vi "PIDControllers (SubVI).vi"(0 "HMI-10HIC200":dbl, 1 "HMI-10LIC200_MA":bool, 2 "BPCS-10LI200":dbl, 3 "HMI-10LIC200-SP":dbl, 5 "HMI-10LIC200-KPID":dbl[](array[numeric]), 7 "HMI-10TIC100-SP":dbl, 9 "BPCS-10TI100":dbl, 11 "HMI-10HIC300":dbl, 12 "HMI-10TIC100_MA":bool, 13 "HMI-10HIC100":dbl, 14 "HMI-10TIC100-KPID":dbl[](array[numeric]), 15 "BPCS-FJ":dbl) -> (4 "BPCS-10Y200":dbl format="%.2f", 6 "BPCS-SIM-TX-ARRAY":dbl[](array[numeric]), 8 "BPCS-10AY300":dbl, 10 "BPCS-10TY100":dbl format="%.2f")   [LabVIEW 2018]
uses:
  <vilib>/addons/control/pid/pid.llb/PID Advanced (DBL).vi
  <vilib>/addons/control/pid/NI_PID_pid.lvlib
panel:
  out "dt out (s)":dbl format="%.3f"
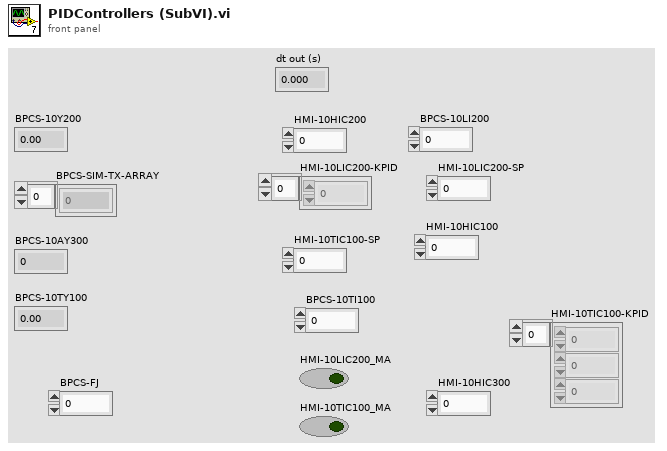
[diagram p1: front panel]
types:
  T1 = cluster{"proportional gain (Kc)":dbl, "integral time (Ti, min)":dbl, "derivative time (Td, min)":dbl}
  T2 = cluster{"HMI-10TIC100-KPID[0]":dbl, "HMI-10TIC100-KPID[1]":dbl, "HMI-10TIC100-KPID[2]":dbl}
  T3 = cluster{"HMI-10LIC200-KPID[0]":dbl, "HMI-10LIC200-KPID[1]":dbl, "HMI-10LIC200-KPID[2]":dbl}
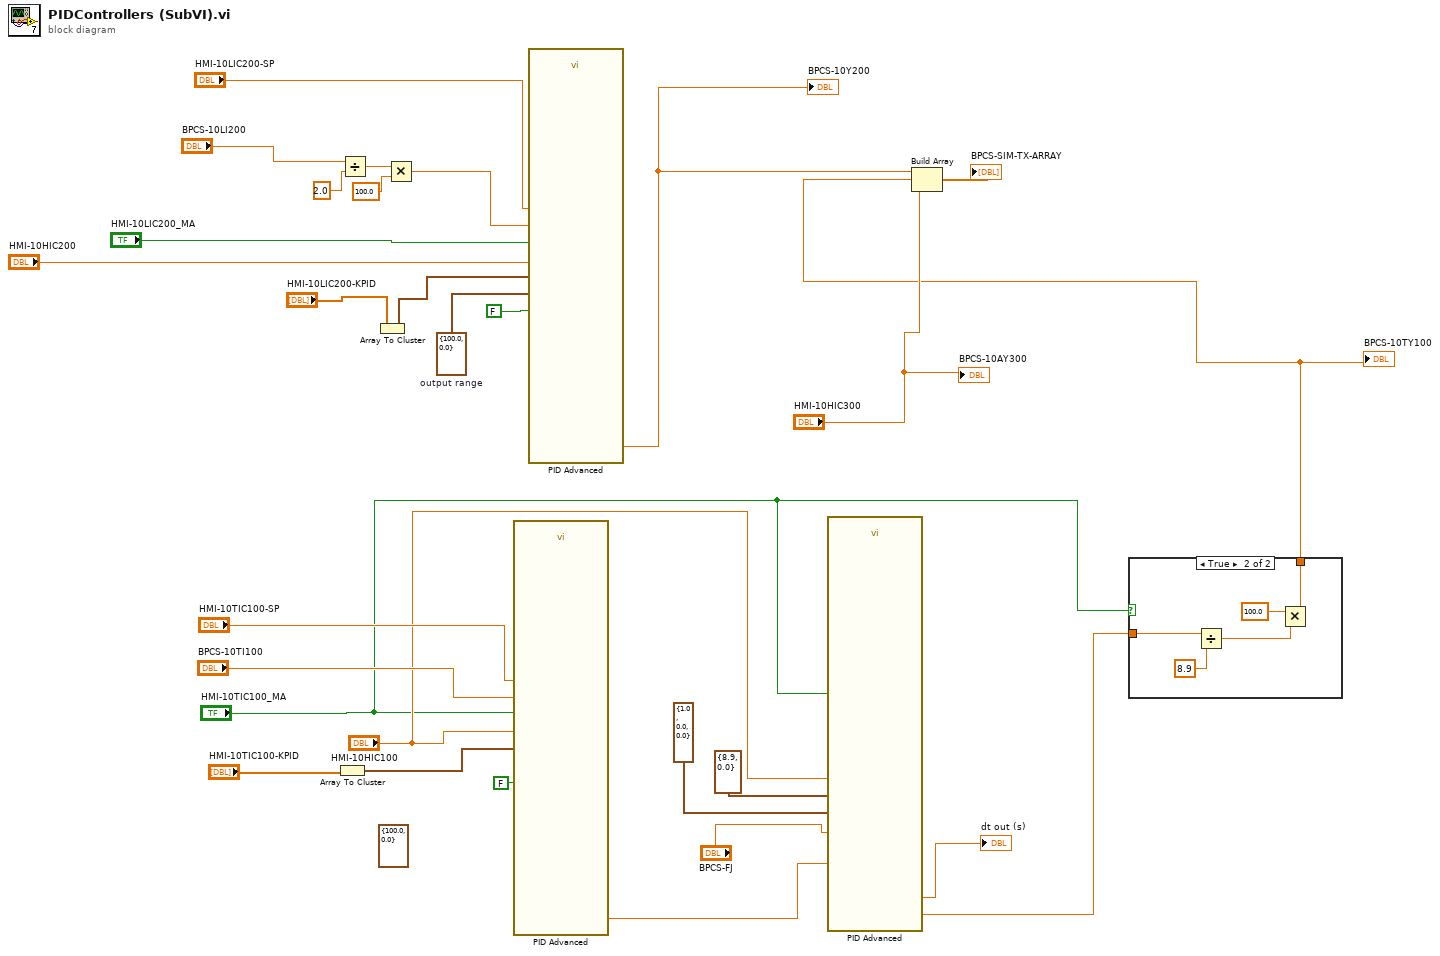
[diagram p0: block diagram]
diagram:
  (unwired) cluster{"output high":dbl, "output low":dbl} {"output high"=100.0, "output low"=0.0} ("output range")
  w19 = cluster{"output high":dbl, "output low":dbl} {"output high"=100.0, "output low"=0.0}  # output range
  n1 = Array To Cluster(array="HMI-10TIC100-KPID") -> (cluster=w20:T2)
  n2 = Divide(x="BPCS-10LI200", y=2.0 ("x")) -> (x/y=w15:dbl)
  n3 = Array To Cluster(array="HMI-10LIC200-KPID") -> (cluster=w18:T3)
  n4 = Multiply(x=w15, y=100.0) -> (x*y=w17:dbl)
  n5 = call-poly <vilib>:"PID Advanced.vi"("setpoint"="HMI-10TIC100-SP", "auto? (T)"="HMI-10TIC100_MA", "manual control"="HMI-10HIC100", "process variable"="BPCS-10TI100", "PID gains"=w20, "reinitialize? (F)"=FALSE) -> ("output"=w7:dbl)  [unwired: 8 in, 1 out]
  n6 = call-poly <vilib>:"PID Advanced.vi"("setpoint"="HMI-10LIC200-SP", "output range"=w19, "auto? (T)"="HMI-10LIC200_MA", "manual control"="HMI-10HIC200", "process variable"=w17, "PID gains"=w18, "reinitialize? (F)"=FALSE) -> ("output"=w11:dbl)  [unwired: 7 in, 1 out]
  "BPCS-10Y200" <- w11
  n7 = call-poly <vilib>:"PID Advanced.vi"("setpoint"=w7, "output range"=cluster{"setpoint high":dbl, "setpoint low":dbl} {"setpoint high"=8.9, "setpoint low"=0.0} ("setpoint range"), "auto? (T)"="HMI-10TIC100_MA", "manual control"="HMI-10HIC100", "process variable"="BPCS-FJ", "PID gains"=T1 {"proportional gain (Kc)"=1.0, "integral time (Ti, min)"=0.0, "derivative time (Td, min)"=0.0}) -> ("output"=w3:dbl, "dt out (s)"=→"dt out (s)":dbl)  [unwired: 8 in]
  n8 = case shown="True" "HMI-10TIC100_MA" {
    tunnel: w3 -> [w30 w32]
    tunnel: [w30 w31] -> w2
    frame False {
    }
    frame True {
      n9 = Divide(x=w32, y=8.9) -> (x/y=w35:dbl)
      n10 = Multiply(x=100.0, y=w35) -> (x*y=w31:dbl)
    }
  }
  "BPCS-10TY100" <- w2
  n11 = Build Array(w11, w2, "HMI-10HIC300") -> (→"BPCS-SIM-TX-ARRAY":dbl[])
  "BPCS-10AY300" <- "HMI-10HIC300"
